vi "CheckLoopError.vi"(0 "object in":refnum<class "Application.lvclass">, 1 "error to process":errorcluster, 3 "Ignore Errors":i32[](array[numeric]), 4 "Exit on Error? (F)":bool) -> (14 "object out":refnum<class "Application.lvclass">, 17 "Error?":bool)   [LabVIEW 2021, in "Application.lvclass"]
uses:
  Application.lvclass
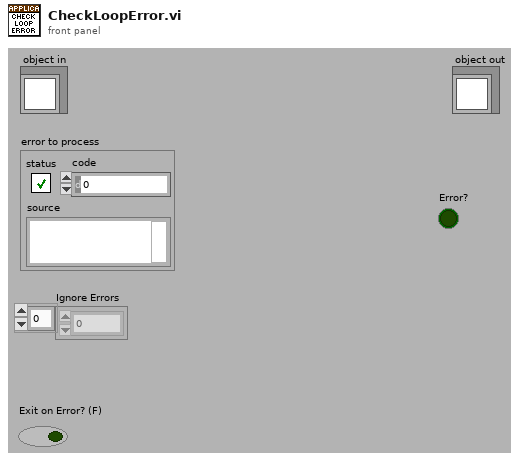
[diagram p1: front panel]
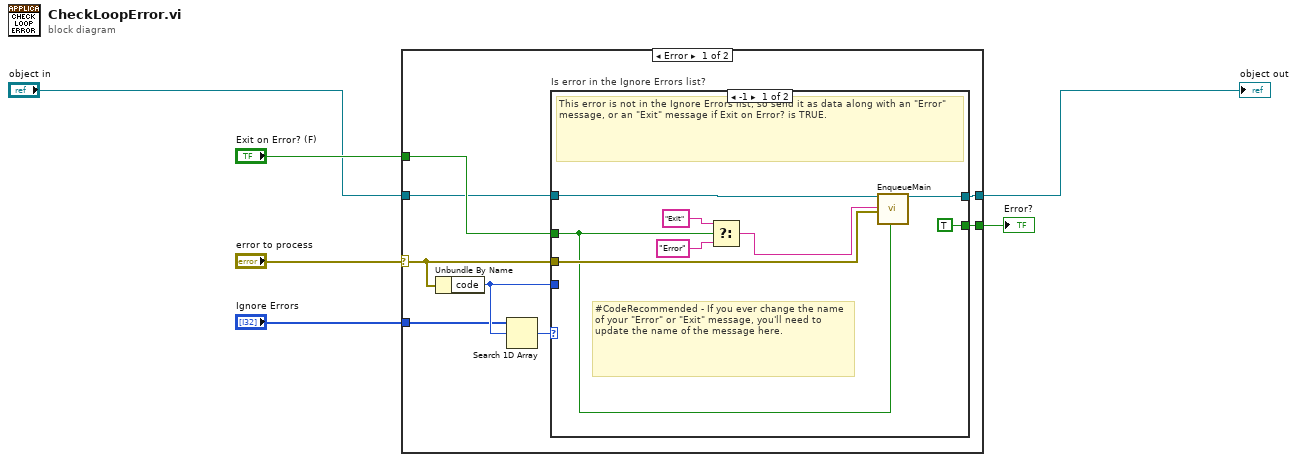
[diagram p0: block diagram]
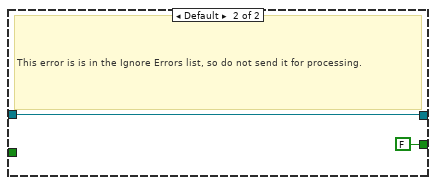
[diagram p2: hidden frame]
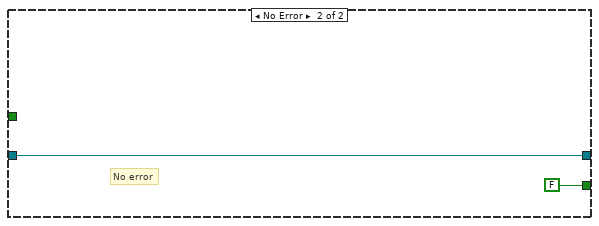
[diagram p3: hidden frame]
diagram:
  n1 = case shown="Error" "error to process" {
    selector: "error to process" -> [w12 _]
    tunnel: "Ignore Errors" -> [w11 _]
    tunnel: [w10 FALSE] -> w4
    tunnel: "Exit on Error? (F)" -> [w9 _]
    tunnel: "object in" -> [w8 w25]
    tunnel: [w7 w25] -> w1
    frame Error {
      n2 = Unbundle By Name(w12) -> ("code"=w13:i32)
      n3 = Search 1D Array(1D array=w11, element=w13) -> (index of element=w14:i32)  [unwired: 1 in]
      n4 = case "Is error in the Ignore Errors list?" shown="-1" w14 {
        tunnel: w12 -> [w17 _]
        tunnel: w13 -> [_ _]
        tunnel: [TRUE FALSE] -> w10
        tunnel: w9 -> [w16 _]
        tunnel: w8 -> [w19 w23]
        tunnel: [w15 w23] -> w7
        frame -1 {
          # "#CodeRecommended - If you ever change the name of your \"Error\" or \"Exit\" message, you'll need to update the name of the message here."
          # "This error is not in the Ignore Errors list, so send it as data along with an \"Error\" message, or an \"Exit\" message if Exit on Error? is TRUE."
          n5 = Select(t="Exit" ("Message"), s=w16, f="Error" ("Message")) -> (s? t:f=w18:string)
          n6 = call-dynamic "EnqueueMain.vi"("object in"=w19, "Message"=w18, "Message Data"=w17, "Priority Message? (F)"=w16) -> ("object out"=w15:refnum<class "Application.lvclass">)  [unwired: 14 in, 1 out]
        }
        frame Default {
          # "This error is is in the Ignore Errors list, so do not send it for processing."
        }
      }
    }
    frame No Error {
      # "No error"
    }
  }
  "object out" <- w1
  "Error?" <- w4
